vi "nanocal -- nuclear schottky fit V3.vi"() -> ()   [LabVIEW 2020] (continued)
                  n124 = for {
                    tunnel: w252 -> [w257]
                    tunnel: w251 -> [w259]
                    tunnel: w250 -> [w258]
                    tunnel: w246 -> [w254] mode=indexing
                    tunnel: [w262] -> w248 mode=indexing
                    tunnel: [w254] -> w247 mode=indexing
                    tunnel: w237 -> [w255]
                    tunnel: w236 -> [w256]
                    n125 = Insert Into Map(map in=w255, key=w256, value=w254) -> (map out=w253:map{T1, dbl})  [unwired: 2 out]
                    n126 = local read "weighting"() -> (w261:T5)
                    n127 = call "nanocal -- nuclear schottky goodness V5.vi"("action"=3-lorentzian-heat-response_action."onlygrads", "parameters IN"=w253, "weighting strategy"=w261, "dz/dω IN (V)"=w257, "Voltage IN (V)"=w259, "ω (rad/sec)"=w258) -> ("R norm"=w264:dbl, "G"=w263:dbl)  [unwired: 2 in, 2 out]
                    n128 = Divide(x=w263, y=w264) -> (x/y=w262:dbl)
                  }
                  n129 = Look In Map(map=w237, key=w236) -> (value=w235:dbl)  [unwired: 1 in, 1 out]
                  n130 = Look In Map(map=w243, key=w236) -> (value=w238:u32)  [unwired: 1 in, 1 out]
                  n131 = Look In Map(map=w242, key=w236) -> (value=w240:i32)  [unwired: 1 in, 1 out]
                  n132 = call "replace plot - plot ref - V2.vi"("Plot ref in"=w234, "Array X IN"=w247, "Array Y IN"=w248, "plot index"=w240, "cursor action"=cursor_action."write") -> ("Plot ref out"=w245:refnum<vi>)  [unwired: 11 in, 3 out]
                  n133 = call "replace cursor - plot ref - V2.vi"("Plot ref in"=w234, "new X"=w235, "cursor index"=w240, "cursor action"=cursor_action."write", "Color Box"=w238, "cursor state"=cursor_sate."colored") -> ()  [unwired: 10 in, 4 out]
                  n134 = call "replace plot - plot ref - V2.vi"("Plot ref in"=w245, "plot index"=w240, "cursor action"=cursor_action."set color", "Color Box"=w238) -> ()  [unwired: 12 in, 4 out]
                }
              }
              frame "2d plots " {
                n135 = for {
                  tunnel: w276 -> [w286]
                  tunnel: w275 -> [w285]
                  tunnel: w274 -> [w284]
                  tunnel: w273 -> [w283]
                  tunnel: w272 -> [w282]
                  tunnel: w271 -> [w281] mode=indexing
                  tunnel: w270 -> [w280]
                  tunnel: w269 -> [w279]
                  shift-right: [w277] -> w266
                  shift-left: "{ " -> [w278]
                  n136 = for {
                    tunnel: w286 -> [w305]
                    tunnel: w285 -> [w307]
                    tunnel: w284 -> [w306]
                    tunnel: w280 -> [w288] mode=indexing
                    tunnel: w281 -> [w287]
                    tunnel: w283 -> [w303]
                    tunnel: w282 -> [w304]
                    tunnel: w279 -> [w302]
                    shift-right: [w298] -> w277
                    shift-left: w278 -> [w299]
                    w291 = " ,     "
                    w297 = i16 12 ("precision (6)")
                    n137 = Insert Into Map(map in=w303, key=w304, value=w288) -> (map out=w300:map{T1, dbl})  [unwired: 2 out]
                    n138 = Insert Into Map(map in=w300, key=w302, value=w287) -> (map out=w301:map{T1, dbl})  [unwired: 2 out]
                    n139 = local read "weighting"() -> (w309:T5)
                    n140 = Number To Fractional String(number=w288, precision (6)=w297) -> (F-format string=w295:string)  [unwired: 2 in]
                    n141 = call "nanocal -- nuclear schottky goodness V5.vi"("action"=3-lorentzian-heat-response_action."onlygrads", "parameters IN"=w301, "weighting strategy"=w309, "dz/dω IN (V)"=w305, "Voltage IN (V)"=w307, "ω (rad/sec)"=w306) -> ("R norm"=w311:dbl, "G"=w310:dbl)  [unwired: 2 in, 2 out]
                    n142 = Number To Fractional String(number=w287, precision (6)=w297) -> (F-format string=w294:string)  [unwired: 2 in]
                    n143 = Divide(x=w310, y=w311) -> (x/y=w296:dbl)
                    n144 = Number To Fractional String(number=w296, precision (6)=w297) -> (F-format string=w293:string)  [unwired: 2 in]
                    n145 = Concatenate Strings(w299, "{    ", w295, w291, w294, w291, w293, " } , ", "\r") -> (w298:string)
                  }
                }
                n146 = Concatenate Strings(w266, " }   ") -> (→"2dplots":string)
              }
            }
          }
          frame "action: gradient step" {
            w320 = 6.283185307179586
            w325 = FALSE ("newton pause")
            n147 = call "nanocal -- publish -- freq scan V2.vi"("publisher action"=publisher_action."get") -> ("dz/dω out (V)"=w322:cdb[], "z out (V)"=w317:cdb[], "ω out (Hz)"=w321:dbl[])  [unwired: 8 in]
            n148 = local write "newton pause"(w325) -> ()
            n149 = Generate User Event(user event=w324, event data cluster="action: new sweep" ("event data")) -> ()  [unwired: 2 in, 2 out]
            n150 = Divide(x=w322, y=w320) -> (x/y=w318:cdb[])
            n151 = Multiply(x=w321, y=w320) -> (x*y=w316:dbl[])
            n152 = for {
              N: "# steps" -> [_]
              tunnel: [TRUE ("newton pause")] -> w326
              tunnel: w325 -> [_]
              shift-right: [w362] -> _
              shift-left: w323 -> [w362]
              tunnel: w318 -> [w345]
              tunnel: w317 -> [w344]
              tunnel: w316 -> [w343]
              stop <- w370 stop-if-true
              (unwired) 3-lorentzian-parameters."κ0" ("Plost: sweep window")
              (unwired) 3-lorentzian-parameters."τC" ("Plost: sweep window")
              (unwired) 3-lorentzian-parameters."τN" ("Plost: sweep window")
              (unwired) 3-lorentzian-parameters."τS" ("Plost: sweep window")
              (unwired) 3-lorentzian-parameters."τ1" ("Plost: sweep window")
              (unwired) 3-lorentzian-parameters."ζ" ("Plost: sweep window")
              w340 = T1[] [enum."ζ", enum."τ1", enum."τS", enum."τN", enum."τC", enum."κ0"] items=["ζ", "τ1", "τS", "τN", "τC", "κ0", "m1", "m2", "m3", "T (K)", "B (T)", "θ (deg)", "side (S|R)", "change (B|T)"]
              n153 = local read "newton pause"() -> (w370:bool)
              n154 = local read "T1"() -> (w375:dbl)
              n155 = local read "τS"() -> (w374:dbl)
              n156 = local read "τN"() -> (w373:dbl)
              n157 = local read "τC"() -> (w372:dbl)
              n158 = local read "κ0"() -> (w371:dbl)
              n159 = local read "ζ"() -> (w376:dbl)
              n160 = Build Array(w376, w375, w374, w373, w372, w371) -> (w347:dbl[])
              n161 = for {
                shift-right: [w399] -> w346
                shift-left: map{T1, dbl} {} ("Map IN") -> [w400]
                tunnel: w340 -> [w397] mode=indexing
                tunnel: w347 -> [w398] mode=indexing
                tunnel: [w397] -> w339 mode=indexing
                n162 = Insert Into Map(map in=w400, key=w397, value=w398) -> (map out=w399:map{T1, dbl})  [unwired: 2 out]
              }
              n163 = local read "newton action"() -> (w331:T6)
              n164 = local read "factor"() -> (w329:dbl)
              n165 = local read "weighting"() -> (w330:T5)
              n166 = local read "what"() -> (w334:cluster{"scaling":dbl, "what":T1}[])
              n167 = call "nanocal -- nuclear schottky goodness V5.vi"("action"=w331, "parameters IN"=w346, "weighting strategy"=w330, "dz/dω IN (V)"=w345, "Voltage IN (V)"=w344, "ω (rad/sec)"=w343) -> ("R norm"=w337:dbl, "G"=w338:dbl, "R(ω) out"=w342:cdb[], "dG / d log α   OUT"=w341:map{T1, dbl})  [unwired: 2 in]
              n168 = Complex To Re/Im(x + iy=w342) -> (x=w359:dbl[], y=w358:dbl[])
              n169 = control-ref of="Plot: sweep window"() -> (w361:refnum<vi>)
              n170 = call "3-lorentzian-heat-response -- V4.vi"("action"=3-lorentzian-heat-response_action."calc m1m2m3", "Map IN"=w346) -> ("Map OUT"=w350:map{T1, dbl})  [unwired: 7 in, 2 out]
              n171 = for {
                tunnel: w339 -> [w395] mode=indexing
                shift-right: [w396] -> _
                shift-left: w341 -> [w396]
                tunnel: [w391] -> w335 mode=indexing
                tunnel: w334 -> [w394] mode=indexing
                tunnel: w329 -> [w390]
                tunnel: [w389] -> w333 mode=indexing
                n172 = Unbundle By Name(w394) -> ("scaling"=w392:dbl)
                n173 = Look In Map(map=w396, key=w395) -> (value=w391:dbl)  [unwired: 1 in, 1 out]
                n174 = Compound Arithmetic op=MULTIPLY(w392, w390, -1.0 ("index"), w391) -> (w389:dbl)
              }
              n175 = local read "cursor x selector"() -> (w355:map{T1, dbl})
              n176 = local read "X selector"() -> (w354:T1)
              n177 = local read "cursor index map"() -> (w351:map{T1, i32})
              n178 = call "replace plot - plot ref - V2.vi"("Plot ref in"=w361, "Array X IN"=w359, "Array Y IN"=w358, "plot index"=enum16{"data R(ω)", "fit R(ω)"}."fit R(ω)" ("Plost: sweep window"), "cursor action"=cursor_action."write") -> ()  [unwired: 11 in, 4 out]
              n179 = local read "T (K)"() -> (w353:dbl)
              n180 = control-ref of="Plot:  colors"() -> (w356:refnum<vi>)
              n181 = Look In Map(map=w355, key=w354, default value=w353) -> (value=w352:dbl)  [unwired: 1 out]
              n182 = Exponential(1:w333) -> (0:w332:dbl[])
              n183 = for {
                tunnel: w352 -> [w408]
                tunnel: w356 -> [w407]
                tunnel: w340 -> [w403] mode=indexing
                tunnel: w351 -> [w405]
                shift-right: [w402] -> _
                shift-left: w350 -> [w402]
                n184 = Look In Map(map=w402, key=w403) -> (value=w401:dbl)  [unwired: 1 in, 1 out]
                n185 = Look In Map(map=w405, key=w403) -> (value=w404:i32)  [unwired: 1 in, 1 out]
                n186 = call "replace cursor - plot ref - V2.vi"("Plot ref in"=w407, "new X"=w408, "new  Y"=w401, "cursor index"=w404, "cursor action"=cursor_action."write") -> ()  [unwired: 11 in, 4 out]
              }
              n187 = Index Array(array=w332, index #1=3-lorentzian-parameters."ζ" ("Plost: sweep window"), index #2=3-lorentzian-parameters."τ1" ("Plost: sweep window"), index #3=3-lorentzian-parameters."τS" ("Plost: sweep window"), index #4=3-lorentzian-parameters."τN" ("Plost: sweep window"), index #5=3-lorentzian-parameters."τC" ("Plost: sweep window"), index #6=3-lorentzian-parameters."κ0" ("Plost: sweep window")) -> (element #1=w383:dbl, element #2=w382:dbl, element #3=w381:dbl, element #4=w380:dbl, element #5=w379:dbl, element #6=w377:dbl)
              n188 = Divide(x=w338, y=w337) -> (x/y=w336:dbl)
              n189 = local write "logarithmic derivatives"(w335) -> ()
              n190 = local write "goodness"(w336) -> ()
              n191 = Multiply(x=w383, y=w376) -> (x*y=w388:dbl)
              n192 = Multiply(x=w382, y=w375) -> (x*y=w387:dbl)
              n193 = Multiply(x=w381, y=w374) -> (x*y=w386:dbl)
              n194 = Multiply(x=w380, y=w373) -> (x*y=w385:dbl)
              n195 = Multiply(x=w379, y=w372) -> (x*y=w384:dbl)
              n196 = Multiply(x=w377, y=w371) -> (x*y=w378:dbl)
              n197 = local write "τN"(w385) -> ()
              n198 = local write "τC"(w384) -> ()
              n199 = local write "τS"(w386) -> ()
              n200 = local write "κ0"(w378) -> ()
              n201 = local write "T1"(w387) -> ()
              n202 = local write "ζ"(w388) -> ()
            }
            n203 = local write "newton pause"(w326) -> ()
          }
          frame "action: uco" {
            (unwired) 3-lorentzian-parameters."κ0" ("Plost: sweep window")
            n204 = Generate User Event(user event=w431, event data cluster="action: new sweep" ("event data")) -> ()  [unwired: 2 in, 2 out]
            n205 = local read "T1"() -> (w423:dbl)
            n206 = local read "τN"() -> (w421:dbl)
            n207 = local read "τC"() -> (w420:dbl)
            n208 = local read "κ0"() -> (w419:dbl)
            n209 = local read "τS"() -> (w422:dbl)
            n210 = local read "ζ"() -> (w424:dbl)
            n211 = call "3-lorentzian-parameters - manage.vi"("ζ"=w424, "T1"=w423, "τS"=w422, "τN"=w421, "τC"=w420, "κ0"=w419, "parameters"=3-lorentzian-parameters_--_action."to array") -> ("parameter array OUT"=w417:dbl[])  [unwired: 6 in, 6 out]
            n212 = Natural Logarithm(1:w417) -> (0:w429:dbl[])
            n213 = vi-ref "nanocal -- nuclear schottky goodness -- for UCO -- V3.vi"() -> (w430:refnum<vi>)
            n214 = call-poly <vilib>:"Unconstrained Optimization.vi"("function data"=T18 variant, "objective function"=w430, "start"=w429) -> ("f(minimum)"=w427:dbl, "minimum"=w428:dbl[])  [unwired: 5 in, 2 out]
            n215 = Exponential(1:w427) -> (0:w426:dbl)
            n216 = Exponential(1:w428) -> (0:w416:dbl[])
            n217 = call "3-lorentzian-parameters - manage.vi"("parameter array"=w416, "parameters"=3-lorentzian-parameters_--_action."to parameters") -> ("ζ OUT"=w415:dbl, "T1 OUT"=w414:dbl, "τS  OUT"=w413:dbl, "τN  OUT"=w412:dbl, "τC  OUT"=w411:dbl, "κ0  OUT"=w410:dbl)  [unwired: 11 in, 1 out]
            n218 = local write "goodness"(w426) -> ()
            n219 = local write "T1"(w414) -> ()
            n220 = local write "τN"(w412) -> ()
            n221 = local write "τC"(w411) -> ()
            n222 = local write "κ0"(w410) -> ()
            n223 = local write "τS"(w413) -> ()
            n224 = local write "ζ"(w415) -> ()
          }
          frame "action: parse string" {
            n225 = local read "String"() -> (w451:string)
            n226 = call "string parse mathematica assosiated array.vi"("derivative"=mathematica_string_map_action."parse string", "String in"=w451) -> ("Map OUT"=w445:map{T1, dbl})  [unwired: 8 in, 1 out]
            n227 = Generate User Event "action User Event"(user event=w449, event data cluster="action: update state of selectors" ("event data")) -> (user event out=w433:refnum<user-event>)  [unwired: 2 in, 1 out]
            n228 = Look In Map(map=w445, key=3-lorentzian-parameters."ζ" ("Plost: sweep window")) -> (value=w440:dbl)  [unwired: 1 in, 1 out]
            n229 = Look In Map(map=w445, key=3-lorentzian-parameters."τ1" ("Plost: sweep window")) -> (value=w439:dbl)  [unwired: 1 in, 1 out]
            n230 = Look In Map(map=w445, key=3-lorentzian-parameters."τS" ("Plost: sweep window")) -> (value=w438:dbl)  [unwired: 1 in, 1 out]
            n231 = Look In Map(map=w445, key=3-lorentzian-parameters."τN" ("Plost: sweep window")) -> (value=w437:dbl)  [unwired: 1 in, 1 out]
            n232 = Look In Map(map=w445, key=3-lorentzian-parameters."τC" ("Plost: sweep window")) -> (value=w436:dbl)  [unwired: 1 in, 1 out]
            n233 = Look In Map(map=w445, key=3-lorentzian-parameters."κ0" ("Plost: sweep window")) -> (value=w435:dbl)  [unwired: 1 in, 1 out]
            n234 = local write "ζ"(w440) -> ()
            n235 = local write "T1"(w439) -> ()
            n236 = local write "τS"(w438) -> ()
            n237 = local write "τN"(w437) -> ()
            n238 = local write "τC"(w436) -> ()
            n239 = local write "κ0"(w435) -> ()
            n240 = Generate User Event "action User Event"(user event=w433, event data cluster="action: replot colors" ("event data")) -> ()  [unwired: 2 in, 2 out]
          }
          frame "action: read mathematica string" {
            w455 = T19[] [enum."get T", enum."get B", enum."get deg", enum."get side", enum."get change"] items=["rewrite", "parse", "force pattern", "uniquenum", "get T", "get B", "get ind", "get deg", "get name", "get folder", "get extension", "get basename", "get side", "get change"]
            w457 = map{T1, T19} {}  # Size: 0
            w456 = T1[] [enum."T (K)", enum."B (T)", enum."θ (deg)", enum."side (S|R)", enum."change (B|T)"] items=["ζ", "τ1", "τS", "τN", "τC", "κ0", "m1", "m2", "m3", "T (K)", "B (T)", "θ (deg)", "side (S|R)", "change (B|T)"]
            w466 = map{T1, dbl} {}  # Size: 0
            w452 = set{dbl} {}  # Size: 0
            w469 = map{i32, map{T1, dbl}} {}  # Size: 0
            w470 = map{i32, string} {}  # Size: 0
            n241 = Generate User Event(user event=w462, event data cluster="action: update enums" ("event data")) -> ()  [unwired: 2 in, 2 out]
            n242 = for {
              shift-right: [w478] -> w454
              shift-left: w457 -> [w479]
              tunnel: w456 -> [w477] mode=indexing
              tunnel: w455 -> [w476] mode=indexing
              n243 = Insert Into Map(map in=w479, key=w477, value=w476) -> (map out=w478:map{T1, T19})  [unwired: 2 out]
            }
            n244 = call "string parse mathematica list assosiated array.vi"("derivative"=3-lorentzian-heat-response_action."parse string", "string IN"="string IN") -> ("Map OUT"=w471:map{i32, map{T1, dbl}})  [unwired: 8 in, 1 out]
            n245 = List Folder(path="folder", pattern="file pattern") -> (filenames=w472:string[])  [unwired: 2 in, 3 out]
            n246 = for {
              tunnel: w472 -> [w482] mode=indexing
              shift-right: [w501] -> w459
              shift-left: w471 -> [w503]
              shift-right: [w499] -> w467
              shift-left: w470 -> [w500]
              shift-right: [w488] -> w460
              shift-left: w469 -> [w489]
              shift-right: [w493] -> w464
              shift-left: w452 -> [w494]
              shift-right: [w495] -> w465
              shift-left: w452 -> [w496]
              tunnel: w466 -> [w485]
              shift-right: [w491] -> w461
              shift-left: w452 -> [w492]
              shift-right: [w487] -> w458
              shift-left: w452 -> [w486]
              tunnel: w454 -> [w484]
              shift-right: [w481] -> w453
              shift-left: w452 -> [w480]
              n247 = for {
                shift-right: [w510] -> w483
                shift-left: w485 -> [w511]
                tunnel: w484 -> [w509] mode=indexing
                tunnel: w482 -> [w507]
                n248 = Unbundle(w509) -> ("key"=w508:T1, "filename-action"=w506:T19)
                n249 = call "filename-manage.vi"("filename-action"=w506, "file name IN"=w507) -> ("number OUT"=w505:dbl)  [unwired: 7 in, 2 out]
                n250 = Insert Into Map(map in=w511, key=w508, value=w505) -> (map out=w510:map{T1, dbl})  [unwired: 2 out]
              }
              n251 = call "filename-manage.vi"("filename-action"=filename-action."get ind", "file name IN"=w482) -> ("number OUT"=w502:dbl)  [unwired: 7 in, 2 out]
              n252 = To Long Integer(number=w502) -> (32bit integer=w490:i32)
              n253 = in-place {
                in-place-border: [w549] -> w498
                in-place-border: w483 -> [w548]
                n254 = in-place-map #1(w503, w490) -> (w547:map{T1, dbl}, w549:bool)  [unwired: 1 in]
                n255 = for {
                  tunnel: w548 -> [w555] mode=indexing
                  shift-right: [w553] -> w546
                  shift-left: w547 -> [w554]
                  n256 = Unbundle(w555) -> ("key"=w552:T1, "number OUT"=w551:dbl)
                  n257 = Insert Into Map(map in=w554, key=w552, value=w551) -> (map out=w553:map{T1, dbl})  [unwired: 2 out]
                }
                n258 = in-place-map #1(w546, LVMapReplaceAction."Modify Entry only if found" ("action")) -> (w501:map{i32, map{T1, dbl}})  [unwired: 2 out]
              }
              n259 = Not(x=w498) -> (.not. x?=w497:bool)
              n260 = case shown="True" w497 {
                tunnel: w500 -> [w518 w545]
                tunnel: [w518 w544] -> w499
                tunnel: w482 -> [_ w543]
                tunnel: w490 -> [_ w519]
                tunnel: w496 -> [w516 w542]
                tunnel: [w516 w541] -> w495
                tunnel: w494 -> [w517 w540]
                tunnel: [w517 w539] -> w493
                tunnel: [w514 w538] -> w491
                tunnel: w492 -> [w514 w537]
                tunnel: w483 -> [_ w522]
                tunnel: w489 -> [w515 w536]
                tunnel: [w515 w535] -> w488
                tunnel: [w513 w534] -> w487
                tunnel: w486 -> [w513 w533]
                tunnel: [w512 w524] -> w481
                tunnel: w480 -> [w512 w523]
                frame False {
                }
                frame True {
                  n261 = Look In Map(map=w522, key=3-lorentzian-parameters."side (S|R)") -> (value=w531:dbl)  [unwired: 1 in, 1 out]
                  n262 = Look In Map(map=w522, key=3-lorentzian-parameters."change (B|T)") -> (value=w525:dbl)  [unwired: 1 in, 1 out]
                  n263 = Look In Map(map=w522, key=3-lorentzian-parameters."B (T)") -> (value=w521:dbl)  [unwired: 1 in, 1 out]
                  n264 = Look In Map(map=w522, key=3-lorentzian-parameters."θ (deg)") -> (value=w520:dbl)  [unwired: 1 in, 1 out]
                  n265 = Look In Map(map=w522, key=3-lorentzian-parameters."T (K)") -> (value=w529:dbl)  [unwired: 1 in, 1 out]
                  n266 = Insert Into Set(10:w531, 11:w533) -> (3:w534:set{dbl})  [unwired: 1 out]
                  n267 = Insert Into Set(10:w529, 11:w537) -> (3:w538:set{dbl})  [unwired: 1 out]
                  n268 = Insert Into Set(10:w521, 11:w542) -> (3:w541:set{dbl})  [unwired: 1 out]
                  n269 = Insert Into Set(10:w520, 11:w540) -> (3:w539:set{dbl})  [unwired: 1 out]
                  n270 = Insert Into Map(map in=w536, key=w519, value=w522) -> (map out=w535:map{i32, map{T1, dbl}})  [unwired: 2 out]
                  n271 = Insert Into Map(map in=w545, key=w519, value=w543) -> (map out=w544:map{i32, string})  [unwired: 2 out]
                  n272 = Insert Into Set(10:w525, 11:w523) -> (3:w524:set{dbl})  [unwired: 1 out]
                }
              }
            }
            "filenames" <- w467
            "Set of B's" <- w465
            "Set of θ's" <- w464
            "Set of T's" <- w461
            "temps&degs" <- w460
            "Set of Sides" <- w458
            "Set of Change" <- w453
            n273 = local write "mathematica thing"(w459) -> ()
          }
          frame "action: empty string from filelist" {
            n274 = local read "file pattern"() -> (w559:string)
            n275 = local read "folder"() -> (w560:path)
            n276 = List Folder(path=w560, pattern=w559) -> (filenames=w558:string[])  [unwired: 2 in, 3 out]
            n277 = for {
              tunnel: w558 -> [w563] mode=indexing
              tunnel: [w562] -> w557 mode=indexing
              n278 = call "filename-manage.vi"("filename-action"=filename-action."get ind", "file name IN"=w563) -> ("number OUT"=w562:dbl)  [unwired: 7 in, 2 out]
            }
            n279 = call "string parse mathematica list assosiated array.vi"("derivative"=3-lorentzian-heat-response_action."create emty string", "array of inds"=w557) -> ("string out"=w556:string)  [unwired: 8 in, 1 out]
            n280 = local write "string OUT"(w556) -> ()
          }
          frame "action: update enums" {
            w568 = map{i32, dbl} {}  # Size: 0
            w572 = map{i32, dbl} {}  # Size: 0
            w578 = map{i32, dbl} {}  # Size: 0
            w586 = map{i32, i32} {}  # Size: 0
            w585 = map{i32, dbl} {}  # Size: 0
            w584 = map{i32, dbl} {}  # Size: 0
            n281 = local read "Set of Change"() -> (w566:set{dbl})
            n282 = Generate User Event(user event=w573, event data cluster="action: update state of selectors" ("event data")) -> ()  [unwired: 2 in, 2 out]
            n283 = for {
              shift-right: [w600] -> w567
              shift-left: w568 -> [w601]
              tunnel: [w598] -> w565 mode=indexing
              tunnel: w566 -> [w597] mode=indexing
              i -> [w599]
              n284 = Number To Decimal String(number=w597) -> (decimal integer string=w598:string)  [unwired: 1 in]
              n285 = Insert Into Map(map in=w601, key=w599, value=w597) -> (map out=w600:map{i32, dbl})  [unwired: 2 out]
            }
            "change lookup" <- w567
            n286 = local read "Set of T's"() -> (w577:set{dbl})
            n287 = local read "Set of Sides"() -> (w570:set{dbl})
            n288 = property on="select change (1T|2B)" class="Ring (strict)"("Strings []"=w565) -> ()  [unwired: 2 in, 2 out]
            n289 = for {
              shift-right: [w611] -> w576
              shift-left: w578 -> [w612]
              tunnel: [w609] -> w575 mode=indexing
              tunnel: w577 -> [w608] mode=indexing
              i -> [w610]
              n290 = Number To Fractional String(number=w608, precision (6)=i16 3) -> (F-format string=w609:string)  [unwired: 2 in]
              n291 = Insert Into Map(map in=w612, key=w610, value=w608) -> (map out=w611:map{i32, dbl})  [unwired: 2 out]
            }
            "T lookup" <- w576
            n292 = for {
              shift-right: [w605] -> w571
              shift-left: w572 -> [w606]
              tunnel: [w603] -> w569 mode=indexing
              tunnel: w570 -> [w602] mode=indexing
              i -> [w604]
              n293 = Number To Decimal String(number=w602) -> (decimal integer string=w603:string)  [unwired: 1 in]
              n294 = Insert Into Map(map in=w606, key=w604, value=w602) -> (map out=w605:map{i32, dbl})  [unwired: 2 out]
            }
            "Side lookup" <- w571
            n295 = property on="select side (8S|4R)" class="Ring (strict)"("Strings []"=w569) -> ()  [unwired: 2 in, 2 out]
            n296 = local read "temps&degs"() -> (w582:map{i32, map{T1, dbl}})
            n297 = local read "X selector"() -> (w581:T1)
            n298 = local read "filenames"() -> (w583:map{i32, string})
            n299 = property on="select T (K)" class="Ring (strict)"("Strings []"=w575) -> ()  [unwired: 2 in, 2 out]
            n300 = for {
              tunnel: [w639] -> w593 mode=indexing
              tunnel: [w636] -> w591 mode=indexing
              tunnel: [w633] -> w595 mode=indexing
              tunnel: w581 -> [w637]
              tunnel: w583 -> [w635] mode=indexing
              tunnel: w582 -> [w634]
              n301 = Unbundle(w635) -> ("32bit integer"=w633:i32, "file pattern"=w639:string)
              n302 = Look In Map(map=w634, key=w633) -> (value=w638:map{T1, dbl})  [unwired: 1 in, 1 out]
              n303 = Look In Map(map=w638, key=w637) -> (value=w636:dbl)  [unwired: 1 in, 1 out]
            }
            n304 = local read "Set of θ's"() -> (w580:set{dbl})
            n305 = local read "Set of B's"() -> (w579:set{dbl})
            n306 = for {
              shift-right: [w625] -> w590
              shift-left: w585 -> [w626]
              tunnel: [w623] -> w589 mode=indexing
              tunnel: w579 -> [w622] mode=indexing
              i -> [w624]
              n307 = Number To Fractional String(number=w622, precision (6)=i16 3) -> (F-format string=w623:string)  [unwired: 2 in]
              n308 = Insert Into Map(map in=w626, key=w624, value=w622) -> (map out=w625:map{i32, dbl})  [unwired: 2 out]
            }
            "B lookup" <- w590
            n309 = for {
              shift-right: [w631] -> w588
              shift-left: w584 -> [w632]
              tunnel: [w629] -> w587 mode=indexing
              tunnel: w580 -> [w628] mode=indexing
              i -> [w630]
              n310 = Number To Fractional String(number=w628, precision (6)=i16 3) -> (F-format string=w629:string)  [unwired: 2 in]
              n311 = Insert Into Map(map in=w632, key=w630, value=w628) -> (map out=w631:map{i32, dbl})  [unwired: 2 out]
            }
            "θ lookup" <- w588
            n312 = call "array - sorted inexes.vi"("x"=w591) -> ("index array"=w592:i32[])  [unwired: 9 in, 1 out]
            n313 = property on="select B (T)" class="Ring (strict)"("Strings []"=w589) -> ()  [unwired: 2 in, 2 out]
            n314 = property on="select θ (deg)" class="Ring (strict)"("Strings []"=w587) -> ()  [unwired: 2 in, 2 out]
            n315 = for {
              tunnel: w592 -> [w617] mode=indexing
              tunnel: w593 -> [w620]
              tunnel: [w619] -> w594 mode=indexing
              tunnel: w595 -> [w618]
              shift-right: [w613] -> w596
              shift-left: w586 -> [w616]
              i -> [w615]
              n316 = Index Array(array=w620, index=w617) -> (element=w619:string)
              n317 = Index Array(array=w618, index=w617) -> (element=w614:i32)
              n318 = Insert Into Map(map in=w616, key=w615, value=w614) -> (map out=w613:map{i32, i32})  [unwired: 2 out]
            }
            "filesnames lookup" <- w596
            n319 = property on="filenames" class="Ring (strict)"("Strings []"=w594) -> ()  [unwired: 2 in, 2 out]
          }
          frame "action: update constrained file selector" {
            w645 = map{i32, i32} {}  # Size: 0
            n320 = local read "state of all selectors"() -> (w641:map{T1, map{bool, dbl}})
            n321 = local read "temps&degs"() -> (w643:map{i32, map{T1, dbl}})
            n322 = local read "filenames"() -> (w642:map{i32, string})
            n323 = for {
              tunnel: w642 -> [w656] mode=indexing
              tunnel: [w656] -> w644 mode=indexing if=w653
              shift-right: [w655] -> w640
              shift-left: w643 -> [w655]
              tunnel: w641 -> [w652]
              n324 = for {
                tunnel: [w668] -> w654 mode=indexing
                shift-right: [w663] -> _
                shift-left: w656 -> [w663]
                shift-right: [w662] -> _
                shift-left: w655 -> [w662]
                tunnel: w652 -> [w661] mode=indexing
                n325 = Unbundle(w663) -> ("32bit integer"=w667:i32)  [unwired: 1 out]
                n326 = Unbundle(w661) -> ("Plost: sweep window"=w660:T1, "map"=w659:map{bool, dbl})
                n327 = for {
                  tunnel: w659 -> [w671] mode=indexing
                  tunnel: [w670] -> w657
                  tunnel: [w669] -> w658
                  n328 = Unbundle(w671) -> ("ignore side !"=w670:bool, "number OUT"=w669:dbl)
                }
                n329 = Look In Map(map=w662, key=w667) -> (value=w666:map{T1, dbl})  [unwired: 1 in, 1 out]
                n330 = Look In Map(map=w666, key=w660) -> (value=w665:dbl)  [unwired: 1 in, 1 out]
                n331 = Equal?(x=w665, y=w658) -> (x = y?=w664:bool)
                n332 = Or(x=w657, y=w664) -> (x .or. y?=w668:bool)
              }
              n333 = And Array Elements(Boolean array=w654) -> (logical AND=w653:bool)
            }
            n334 = for {
              tunnel: [w686] -> w648 mode=indexing
              tunnel: [w684] -> w646 mode=indexing
              tunnel: [w681] -> w650 mode=indexing
              tunnel: w644 -> [w683] mode=indexing
              tunnel: w640 -> [w682]
              n335 = Unbundle(w683) -> ("32bit integer"=w681:i32, "file pattern"=w686:string)
              n336 = local read "X selector"() -> (w680:T1)
              n337 = Look In Map(map=w682, key=w681) -> (value=w685:map{T1, dbl})  [unwired: 1 in, 1 out]
              n338 = Look In Map(map=w685, key=w680) -> (value=w684:dbl)  [unwired: 1 in, 1 out]
            }
            n339 = call "array - sorted inexes.vi"("x"=w646) -> ("index array"=w647:i32[])  [unwired: 9 in, 1 out]
            n340 = for {
              tunnel: w647 -> [w676] mode=indexing
              tunnel: w648 -> [w679]
              tunnel: [w678] -> w649 mode=indexing
              tunnel: w650 -> [w677]
              shift-right: [w672] -> w651
              shift-left: w645 -> [w675]
              i -> [w674]
              n341 = Index Array(array=w679, index=w676) -> (element=w678:string)
              n342 = Index Array(array=w677, index=w676) -> (element=w673:i32)
              n343 = Insert Into Map(map in=w675, key=w674, value=w673) -> (map out=w672:map{i32, i32})  [unwired: 2 out]
            }
            "constrained filename lookup" <- w651
            n344 = property on="constrained filenames" class="Ring (strict)"("Strings []"=w649) -> ()  [unwired: 2 in, 2 out]
          }
          frame "action: write mathematica string" {
            n345 = local read "mathematica thing"() -> (w691:map{i32, map{T1, dbl}})
            n346 = local read "folder"() -> (w690:path)
            n347 = Build Path(base path=w690, name or relative path="temporarystring.txt") -> (appended path=w689:path)
            n348 = call "string parse mathematica list assosiated array.vi"("derivative"=3-lorentzian-heat-response_action."create string", "Map IN"=w691) -> ("string out"=w687:string)  [unwired: 8 in, 1 out]
            "string OUT" <- w687
            n349 = Write to Text File(file (use dialog)=w689, text=w687) -> ()  [unwired: 2 in, 3 out]
          }
          frame "action: replot colors" {
            # "all -- including kappa0"
            n350 = local read "state of all selectors string"() -> (w704:string)
            n351 = local read "state of all selectors"() -> (w720:map{T1, map{bool, dbl}})
            n352 = local read "new selector names"() -> (w701:map{T1, map{T4, string}})
            n353 = local read "mathematica thing"() -> (w725:map{i32, map{T1, dbl}})
            n354 = local read "X selector"() -> (w694:T1)
            n355 = control-ref of="Plot:  colors"() -> (w696:refnum<vi>)
            n356 = case shown="\"T (K)\", Default" w694 {
              tunnel: ["B (T)" "T (K)"] -> w693
              frame "B (T)" {
              }
              frame "T (K)", Default {
              }
            }
            n357 = Look In Map(map=w701, key=w694) -> (value=w700:map{T4, string})  [unwired: 1 in, 1 out]
            n358 = Array Subset(array=w724, index=0, length=6 ("index")) -> (w722:T1[])
            n359 = Look In Map(map=w700, key=nameformattingitem."nameL") -> (value=w698:string)  [unwired: 1 in, 1 out]
            n360 = call "replace plot - plot ref - V2.vi"("Plot ref in"=w696, "text"=w693, "cursor action"=cursor_action."set Xlabel") -> ("Plot ref out"=w695:refnum<vi>)  [unwired: 13 in, 3 out]
            n361 = Concatenate Strings(w704, w698) -> (w719:string)
            n362 = for {
              tunnel: w725 -> [w764]
              tunnel: w694 -> [w759]
              tunnel: w722 -> [w747] mode=indexing
              tunnel: w720 -> [w760]
              tunnel: w701 -> [w751]
              shift-right: [w755] -> w711
              shift-left: w719 -> [w758]
              tunnel: w704 -> [w756]
              tunnel: [w752] -> w713 mode=indexing
              tunnel: w695 -> [w744]
              n363 = for {
                tunnel: w764 -> [w789] mode=indexing
                tunnel: w747 -> [w788]
                tunnel: [w787] -> w763 mode=indexing if=w781
                tunnel: [w786] -> w762 mode=indexing if=w781
                tunnel: w759 -> [w785]
                tunnel: w760 -> [w784]
                n364 = Unbundle(w789) -> ("Map"=w783:map{T1, dbl})  [unwired: 1 out]
                n365 = for {
                  tunnel: w784 -> [w798] mode=indexing
                  tunnel: w783 -> [w797]
                  tunnel: [w795] -> w782 mode=indexing
                  n366 = Unbundle(w798) -> ("Plost: sweep window"=w796:T1, "map"=w794:map{bool, dbl})
                  n367 = for {
                    tunnel: w794 -> [w801] mode=indexing
                    tunnel: [w800] -> w791
                    tunnel: [w799] -> w792
                    n368 = Unbundle(w801) -> ("ignore side !"=w800:bool, "number OUT"=w799:dbl)
                  }
                  n369 = Look In Map(map=w797, key=w796) -> (value=w793:dbl)  [unwired: 1 in, 1 out]
                  n370 = Equal?(x=w793, y=w792) -> (x = y?=w790:bool)
                  n371 = Or(x=w791, y=w790) -> (x .or. y?=w795:bool)
                }
                n372 = Look In Map(map=w783, key=w785) -> (value=w787:dbl)  [unwired: 1 in, 1 out]
                n373 = Look In Map(map=w783, key=w788) -> (value=w786:dbl)  [unwired: 1 in, 1 out]
                n374 = And Array Elements(Boolean array=w782) -> (logical AND=w781:bool)
              }
              n375 = Look In Map(map=w751, key=w747) -> (value=w749:map{T4, string})  [unwired: 1 in, 1 out]
              n376 = Look In Map(map=w749, key=nameformattingitem."nameL") -> (value=w748:string)  [unwired: 1 in, 1 out]
              n377 = call <vilib>:"Space Constant.vi"() -> ("String"=w757:string)
              n378 = Concatenate Strings(w758, w757, w756, w748) -> (w755:string)
              n379 = call "array - sorted inexes.vi"("x"=w763) -> ("index array"=w761:i32[])  [unwired: 9 in, 1 out]
              n380 = local read "cursor index map"() -> (w745:map{T1, i32})
              n381 = for {
                tunnel: w763 -> [w780]
                tunnel: w762 -> [w779]
                tunnel: w761 -> [w776] mode=indexing
                tunnel: [w778] -> w754 mode=indexing
                tunnel: [w777] -> w753 mode=indexing
                n382 = Index Array(array=w780, index=w776) -> (element=w778:dbl)
                n383 = Index Array(array=w779, index=w776) -> (element=w777:dbl)
              }
              n384 = local read "color Map"() -> (w746:map{T1, u32})
              n385 = case shown="\"ζ\"..\"τC\", Default" w747 {
                selector: w747 -> [_ w768]
                tunnel: w754 -> [_ w770]
                tunnel: w753 -> [_ w769]
                tunnel: w746 -> [_ w767]
                tunnel: w745 -> [_ w766]
                tunnel: w744 -> [_ w765]
                frame "κ0" {
                }
                frame "ζ".."τC", Default {
                  n386 = Look In Map(map=w766, key=w768) -> (value=w772:i32)  [unwired: 1 in, 1 out]
                  n387 = Look In Map(map=w767, key=w768) -> (value=w771:u32)  [unwired: 1 in, 1 out]
                  n388 = call "replace plot - plot ref - V2.vi"("Plot ref in"=w765, "Array X IN"=w770, "Array Y IN"=w769, "plot index"=w772, "cursor action"=cursor_action."write") -> ("Plot ref out"=w774:refnum<vi>)  [unwired: 11 in, 3 out]
                  n389 = call "replace plot - plot ref - V2.vi"("Plot ref in"=w774, "plot index"=w772, "cursor action"=cursor_action."set color", "Color Box"=w771) -> ()  [unwired: 12 in, 4 out]
                }
              }
              n390 = Bundle(w754, w753) -> (w752:cluster{dbl[], dbl[]})  [unwired: 1 in]
            }
            n391 = Index Array(array=w713, index=0) -> (element=w717:cluster{dbl[], dbl[]})
            n392 = Unbundle(w717) -> (w716:dbl[])  [unwired: 1 out]
            n393 = local read "folder"() -> (w708:path)
            n394 = Concatenate Strings("plotstring", w704, ".dat") -> (w702:string)
            n395 = Build Array(w716) -> (w715:dbl[][])
            n396 = for {
              shift-right: [w741] -> w714
              shift-left: w715 -> [w743]
              tunnel: w713 -> [w740] mode=indexing
              n397 = Unbundle(w740) -> (w742:dbl[])  [unwired: 1 out]
              n398 = Build Array (concatenate)(w743, w742) -> (w741:dbl[][])
            }
            n399 = Build Path(base path=w708, name or relative path=w702) -> (appended path=w707:path)
            n400 = Concatenate Strings(w711, "\r") -> (w709:string)
            n401 = Transpose 2D Array(2D array=w714) -> (transposed array=w712:dbl[][])
            n402 = for {
              shift-right: [w733] -> w706
              shift-left: w709 -> [w732]
              tunnel: w712 -> [w730] mode=indexing
              n403 = for {
                shift-right: [w734] -> w729
                shift-left: "" -> [w739]
                tunnel: w730 -> [w738] mode=indexing
                n404 = Number To Fractional String(number=w738, precision (6)=i16 16) -> (F-format string=w736:string)  [unwired: 2 in]
                n405 = Concatenate Strings(w739, w736, "    ") -> (w734:string)
              }
              n406 = Concatenate Strings(w732, w729, "\r") -> (w733:string)
            }
            n407 = Write to Text File(file (use dialog)=w707, text=w706) -> ()  [unwired: 2 in, 3 out]
          }
          frame "action: update state of selectors" {
            w802 = T1[] [enum."T (K)", enum."B (T)", enum."θ (deg)", enum."side (S|R)"] items=["ζ", "τ1", "τS", "τN", "τC", "κ0", "m1", "m2", "m3", "T (K)", "B (T)", "θ (deg)", "side (S|R)", "change (B|T)"]
            n408 = local read "select change (1T|2B)"() -> (w813:i32)
            n409 = local read "select side (8S|4R)"() -> (w833:i32)
            n410 = local read "ignore change !"() -> (w815:bool)
            n411 = Generate User Event(user event=w807, event data cluster="action: replot colors" ("event data")) -> (user event out=w808:refnum<user-event>)  [unwired: 2 in, 1 out]
            n412 = local read "change lookup"() -> (w814:map{i32, dbl})
            n413 = local read "select θ (deg)"() -> (w839:u16)
            n414 = local read "ignore side !"() -> (w830:bool)
            n415 = local read "Side lookup"() -> (w834:map{i32, dbl})
            n416 = local read "select T (K)"() -> (w835:u16)
            n417 = local read "select B (T)"() -> (w837:u16)
            n418 = local read "ignore B !"() -> (w823:bool)
            n419 = local read "ignore T !"() -> (w828:bool)
            n420 = local read "ignore θ !"() -> (w820:bool)
            n421 = local read "T lookup"() -> (w836:map{i32, dbl})
            n422 = local read "B lookup"() -> (w838:map{i32, dbl})
            n423 = local read "θ lookup"() -> (w840:map{i32, dbl})
            n424 = Look In Map(map=w838, key=w837) -> (value=w822:dbl)  [unwired: 1 in, 1 out]
            n425 = Look In Map(map=w836, key=w835) -> (value=w827:dbl)  [unwired: 1 in, 1 out]
            n426 = Look In Map(map=w840, key=w839) -> (value=w819:dbl)  [unwired: 1 in, 1 out]
            n427 = Look In Map(map=w834, key=w833) -> (value=w829:dbl)  [unwired: 1 in, 1 out]
            n428 = Look In Map(map=w814, key=w813) -> (value=w816:dbl)  [unwired: 1 in, 1 out]
            n429 = node(w823, w822) -> (w821:map{bool, dbl})
            n430 = node(w828, w827) -> (w825:map{bool, dbl})
            n431 = node(w830, w829) -> (w831:map{bool, dbl})
            n432 = node(w820, w819) -> (w817:map{bool, dbl})
            n433 = node(w815, w816) -> (w811:map{bool, dbl})
            n434 = Generate User Event(user event=w808, event data cluster="action: update constrained file selector" ("event data")) -> ()  [unwired: 2 in, 2 out]
            n435 = local read "new selector names"() -> (w805:map{T1, map{T4, string}})
            n436 = node(3-lorentzian-parameters."side (S|R)" ("Plost: sweep window"), w831, 3-lorentzian-parameters."T (K)" ("Plost: sweep window"), w825, 3-lorentzian-parameters."B (T)" ("Plost: sweep window"), w821, 3-lorentzian-parameters."θ (deg)" ("Plost: sweep window"), w817, 3-lorentzian-parameters."change (B|T)" ("Plost: sweep window"), w811) -> (w806:map{T1, map{bool, dbl}})
            "state of all selectors" <- w806
            n437 = for {
              shift-right: [w847] -> _
              shift-left: w806 -> [w847]
              tunnel: w805 -> [w843]
              shift-right: [w846] -> w803
              shift-left: "_" ("event data") -> [w845]
              tunnel: w802 -> [w842] mode=indexing
              n438 = Look In Map(map=w847, key=w842) -> (value=w849:map{bool, dbl})  [unwired: 1 in, 1 out]
              n439 = Look In Map(map=w843, key=w842) -> (value=w841:map{T4, string})  [unwired: 1 in, 1 out]
              n440 = for {
                tunnel: w849 -> [w864] mode=indexing
                tunnel: [w863] -> w848
                tunnel: [w862] -> w844
                n441 = Unbundle(w864) -> ("ignore side !"=w863:bool, "number OUT"=w862:dbl)
              }
              n442 = case shown="False" w848 {
                tunnel: [w860 w861] -> w846
                tunnel: w845 -> [w859 w861]
                tunnel: w844 -> [w856 _]
                tunnel: w841 -> [w852 _]
                frame False {
                  n443 = Look In Map(map=w852, key=nameformattingitem."prec") -> (value=w850:string)  [unwired: 1 in, 1 out]
